vi "DIAdem Enqueue TDM Request.vi"(8 "error in (no error)":errorcluster, 10 "Wait for Completion?":bool=TRUE, 11 "TDM Request":T8={"TDM Path"=path "", "Response queue name"="", "Run String"="", "Optimize Load"={"Load Fields?"=TRUE}, "Custom Fields"=[]}) -> (0 "error out":errorcluster, 2 "timed out?":bool, 3 "Run Data":T1)   [LabVIEW 2011]
uses:
  www/cgi-bin/cgi-lib/View Reports LIB/Load TDM Settings.ctl
  database/Fields/Field Record.ctl
  TDM Queue.ctl
  TDM Run Result.ctl
  database/Fields/Field DataTypes.ctl
  database/Fields/Field NextItem.ctl
  TDMS/TDMS Channel (Sxx).ctl
  TDMS/TDMS Run.ctl
  TDMS/TDMS File.ctl
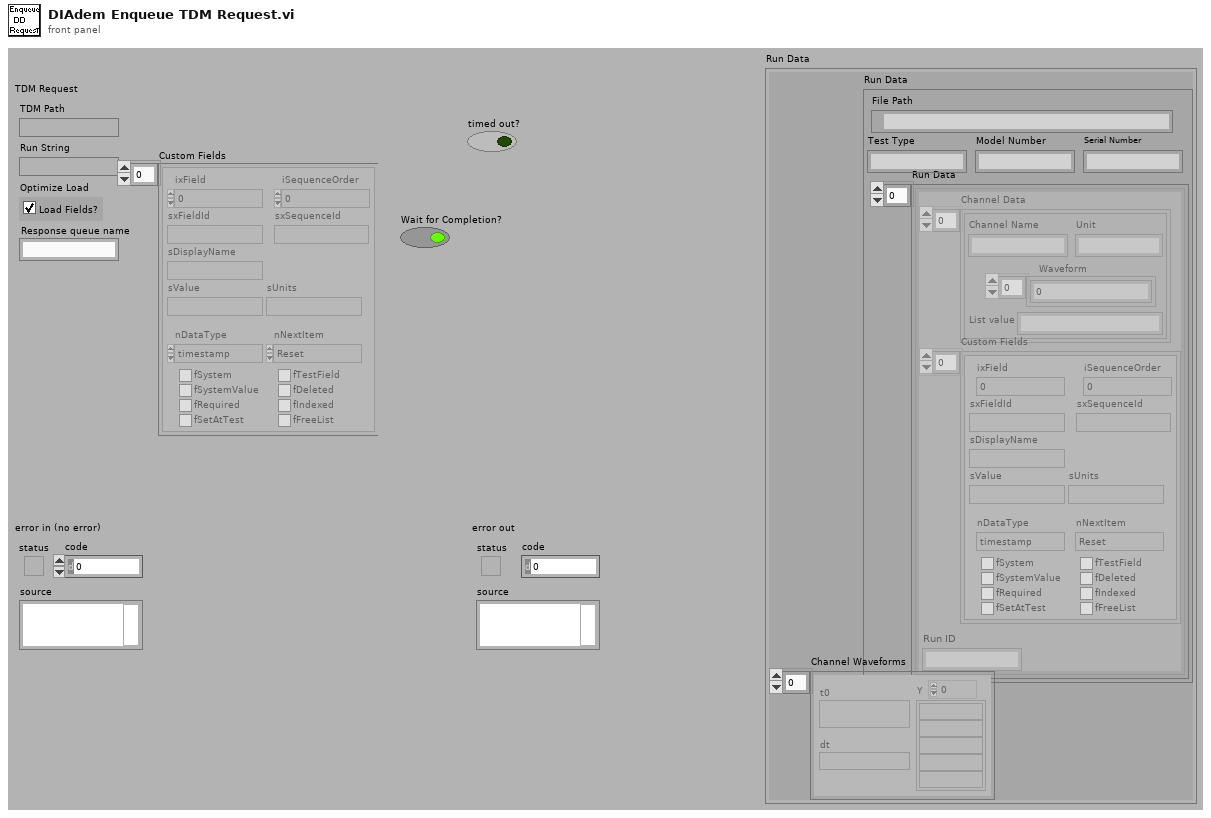
[diagram p1: front panel]
types:
  T1 = typedef "TDM Run Result.ctl" = cluster{"Run Data":T2, "Channel Waveforms":waveform(dbl)[]}
  T2 = typedef "TDMS File.ctl" = cluster{"File Path":path, "Run Data":T3[], "Serial Number":string, "Model Number":string, "Test Type":string}
  T3 = typedef "TDMS Run.ctl" = cluster{"Channel Data":T4[], "Custom Fields":T5[], "Run ID":string}
  T4 = typedef "TDMS Channel (Sxx).ctl" = cluster{"Channel Name":string, "Waveform":dbl[], "Unit":string, "List value":string}
  T5 = typedef "Field Record.ctl" = cluster{"ixField":i32, "iSequenceOrder":i32, "sxFieldId":string, "sxSequenceId":string, "sDisplayName":string, "sValue":string, "sUnits":string, "nDataType":T6, "nNextItem":T7, "fSystem":bool, "fSystemValue":bool, "fRequired":bool, "fSetAtTest":bool, "fTestField":bool, "fDeleted":bool, "fIndexed":bool, "fFreeList":bool}
  T6 = typedef "Field DataTypes.ctl" = enum32{"text", "numeric", "list", "timestamp", "boolean"}
  T7 = typedef "Field NextItem.ctl" = enum32{"Reset", "Retain", "Auto-Increment"}
  T8 = typedef "TDM Queue.ctl" = cluster{"TDM Path":path, "Response queue name":string, "Run String":string, "Optimize Load":T9, "Custom Fields":T5[]}
  T9 = typedef "Load TDM Settings.ctl" = cluster{"Load Fields?":bool}
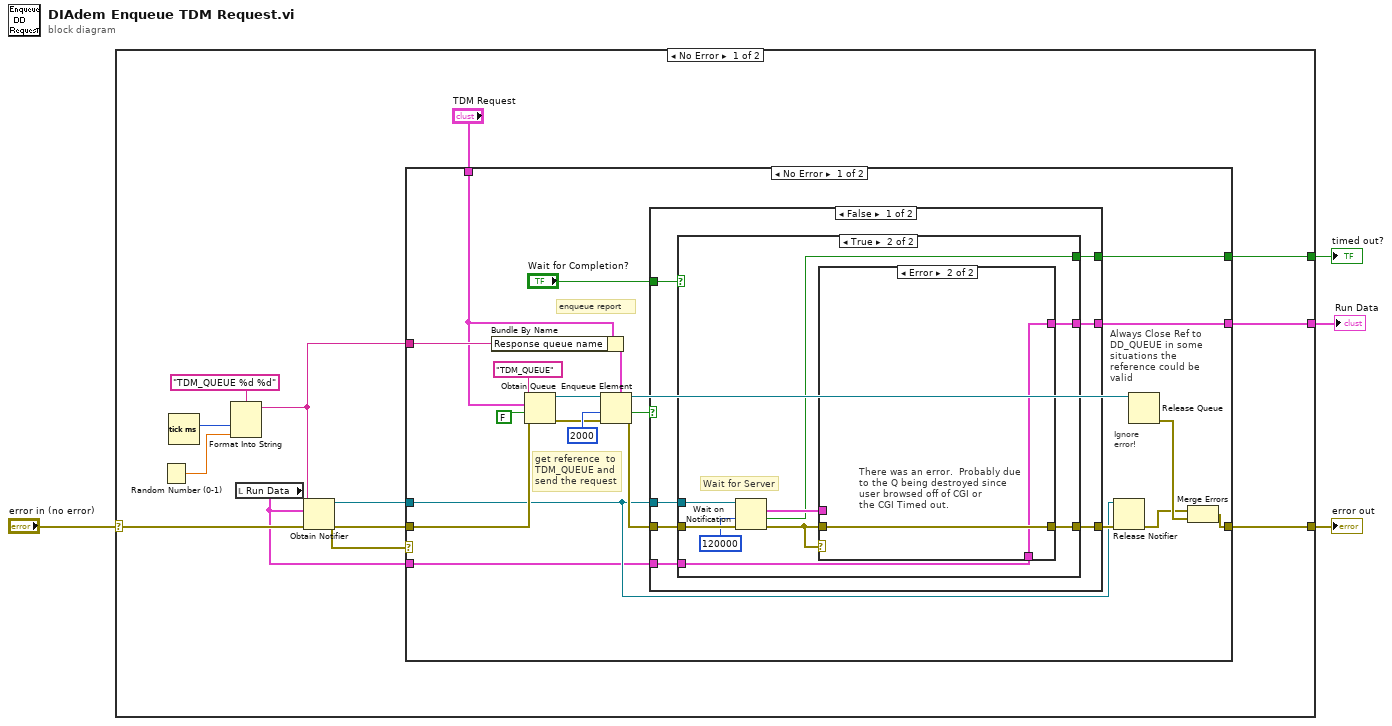
[diagram p0: block diagram]
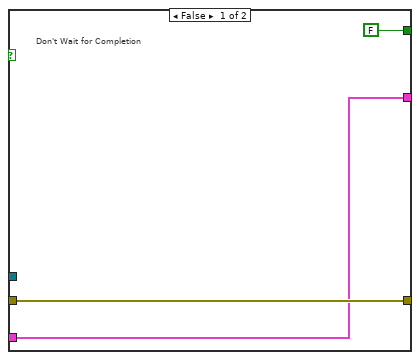
[diagram p2: hidden frame]
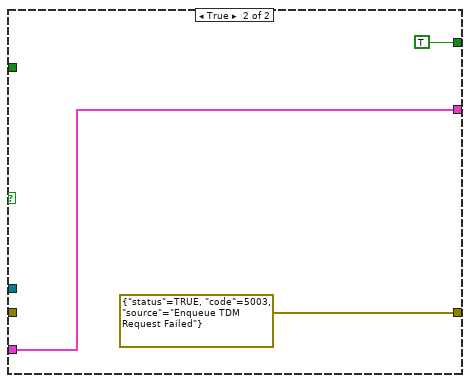
[diagram p4: hidden frame]
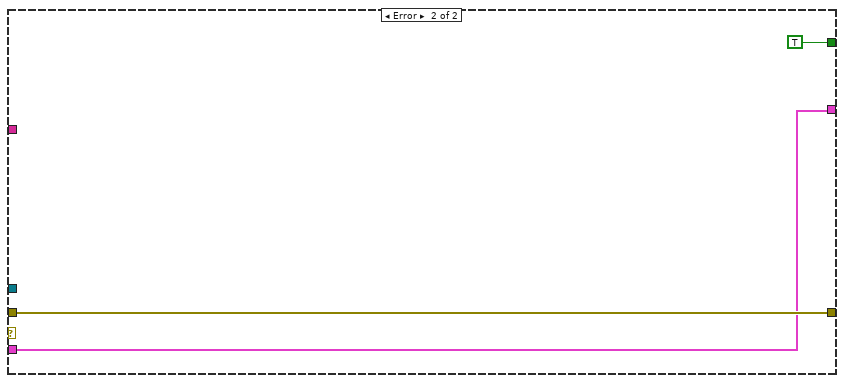
[diagram p5: hidden frame]
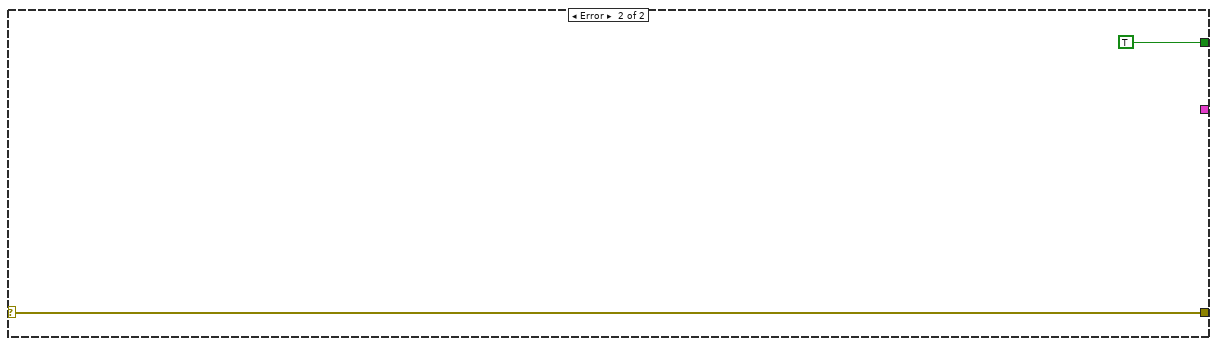
[diagram p6: hidden frame]
diagram:
  n1 = case shown="No Error" "error in (no error)" {
    selector: "error in (no error)" -> [w13 w67]
    tunnel: [w16 _] -> w1
    tunnel: [w15 w67] -> w4
    tunnel: [w14 TRUE ("timed out?")] -> w3
    frame No Error {
      n2 = Random Number (0-1)() -> (number: 0 to 1=w9:dbl)
      n3 = Tick Count (ms)() -> (millisecond timer value=w10:u32)
      n4 = Format Into String(format string="TDM_QUEUE %d %d" ("name (unnamed)"), w10, w9) -> (resulting string=w7:string)  [unwired: 2 in, 1 out]
      n5 = local read "Run Data"() -> (w5:T1)
      n6 = Obtain Notifier(name (unnamed)=w7, notification data type=w5, error in (no error)=w13) -> (notifier out=w6:refnum<notifier>, error out=w8:errorcluster)  [unwired: 1 in, 1 out]
      n7 = case shown="No Error" w8 {
        tunnel: [w37 w64] -> w16
        tunnel: [w23 w66] -> w15
        tunnel: [w26 TRUE ("timed out?")] -> w14
        tunnel: w6 -> [w19 _]
        tunnel: w8 -> [w25 w66]
        tunnel: w7 -> [w22 _]
        tunnel: "TDM Request" -> [w21 _]
        tunnel: w5 -> [w17 w64]
        frame No Error {
          # "Ignore\nerror!"
          # "Always Close Ref to DD_QUEUE in some situations the reference could be valid"
          # "enqueue report"
          # "get reference  to \nTDM_QUEUE and\nsend the request"
          n8 = Bundle By Name(cluster=w21, "Response queue name"=w22) -> (w36:T8)
          n9 = Obtain Queue(name (unnamed)="TDM_QUEUE", element data type=w21, create if not found? (T)=FALSE, error in (no error)=w25) -> (queue out=w29:refnum<queue>, error out=w30:errorcluster)  [unwired: 1 in, 1 out]
          n10 = Enqueue Element(queue=w29, element=w36, timeout in ms (-1)=2000, error in (no error)=w30) -> (queue out=w33:refnum<queue>, timed out?=w31:bool, error out=w32:errorcluster)
          n11 = case shown="False" w31 {
            tunnel: w32 -> [w43 _]
            tunnel: w19 -> [w44 _]
            tunnel: [w42 errorcluster {"status"=TRUE, "code"=5003, "source"="Enqueue TDM Request Failed"} ("error out")] -> w20
            tunnel: "Wait for Completion?" -> [w41 _]
            tunnel: [w40 w61] -> w37
            tunnel: [w39 TRUE ("timed out?")] -> w26
            tunnel: w17 -> [w38 w61]
            frame False {
              n12 = case shown="True" w41 {
                tunnel: w44 -> [_ w51]
                tunnel: w43 -> [w47 w50]
                tunnel: [w47 w56] -> w42
                tunnel: [w45 w55] -> w40
                tunnel: [FALSE ("timed out?") w53] -> w39
                tunnel: w38 -> [w45 w48]
                frame False {
                  # "Don't Wait for Completion"
                }
                frame True {
                  # "Wait for Server"
                  n13 = Wait on Notification(notifier=w51, timeout in ms (-1)=120000, error in (no error)=w50) -> (notification=w54:T1, timed out?=w53:bool, error out=w52:errorcluster)  [unwired: 1 in, 1 out]
                  n14 = case shown="Error" w52 {
                    tunnel: [w58 w60] -> w56
                    tunnel: [w57 w59] -> w55
                    tunnel: w54 -> [w57 _]
                    tunnel: w52 -> [w58 w60]
                    tunnel: w48 -> [_ w59]
                    frame No Error {
                    }
                    frame Error {
                      # "There was an error.  Probably due\nto the Q being destroyed since\nuser browsed off of CGI or\nthe CGI Timed out."
                    }
                  }
                }
              }
            }
            frame True {
            }
          }
          n15 = Release Notifier(notifier=w19, error in (no error)=w20) -> (error out=w18:errorcluster)  [unwired: 1 in, 2 out]
          n16 = Release Queue(queue=w33) -> (error out=w24:errorcluster)  [unwired: 2 in, 2 out]
          n17 = Merge Errors(w18, w24) -> (w23:errorcluster)
        }
        frame Error {
        }
      }
    }
    frame Error {
    }
  }
  "timed out?" <- w3
  "error out" <- w4
  "Run Data" <- w1
